vi "My_DHT11_Labview2.vi"() -> ()   [LabVIEW 2024]
uses:
  <vilib>/Instr/_visa.llb/VISA Configure Serial Port (Instr).vi
panel:
  out "Boolean 2":bool
  out "Temperature":dbl(graph)
  out "Humidity":dbl(knob) scale=0.0..10.0
  out "Boolean":bool
  out "%":dbl(slide) scale=0.0..100.0 scale format="%%%d"
  out "Hum":string
  out "C":dbl(slide) scale=0.0..100.0
  in  "?":bool
  out "Temp":string
  in  "VISA Arduino Uno":refnum<visa-resource-name>
  # "Monitoring Temp&Hum"
  # "Eng. Yahia Gaddal\ngaddal18@gmail.com"
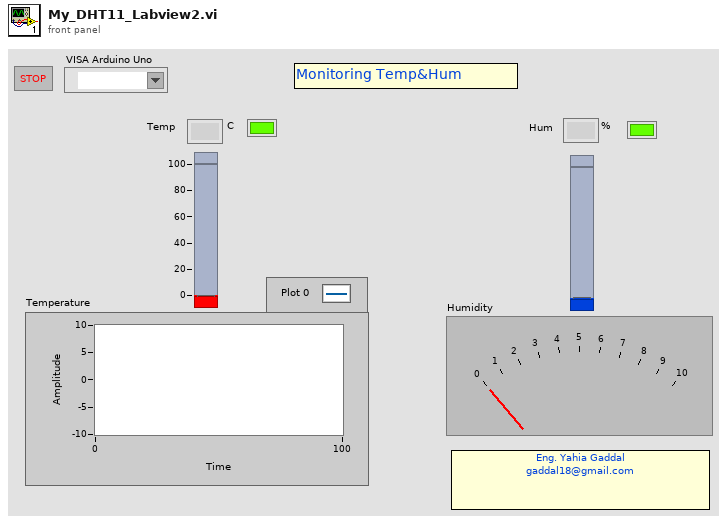
[diagram p1: front panel]
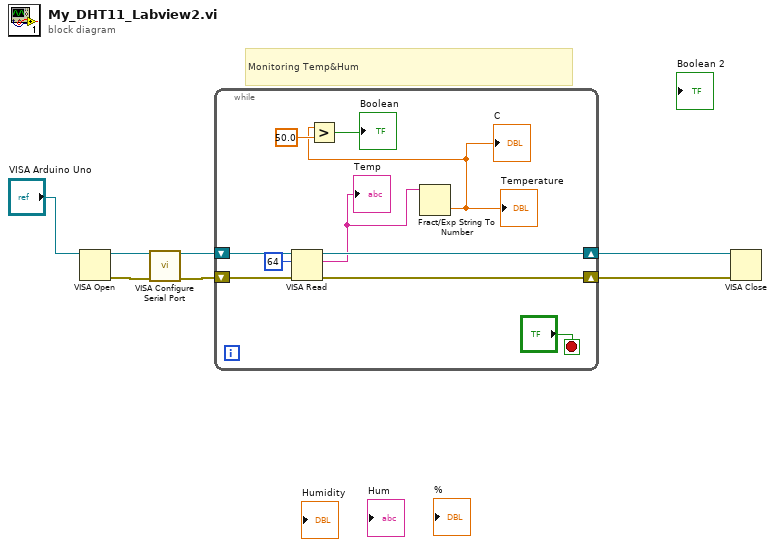
[diagram p0: block diagram]
diagram:
  # "Monitoring Temp&Hum"
  n1 = VISA Open(VISA resource name="VISA Arduino Uno") -> (VISA resource name=w7:refnum<visa-resource-name>, error out=w6:errorcluster)  [unwired: 4 in]
  n2 = call-poly "VISA Configure Serial Port"("VISA resource name"=w7, "error in (no error)"=w6) -> ("VISA resource name out"=w5:refnum<visa-resource-name>, "error out"=w4:errorcluster)  [unwired: 12 in]
  n3 = while {
    shift-right: [w14] -> w3
    shift-left: w5 -> [w17]
    shift-right: [w13] -> w2
    shift-left: w4 -> [w16]
    stop <- "?" stop-if-true
    n4 = VISA Read(VISA resource name=w17, byte count=u32 64, error in (no error)=w16) -> (VISA resource name out=w14:refnum<visa-resource-name>, read buffer=w11:string, error out=w13:errorcluster)  [unwired: 1 out]
    "Temp" <- w11
    n5 = Fract/Exp String To Number(string=w11) -> (number=w8:dbl)  [unwired: 3 in, 1 out]
    "C" <- w8
    "Temperature" <- w8
    n6 = Greater?(x=w8, y=50.0) -> (0:→"Boolean":bool)
  }
  n7 = VISA Close(VISA resource name=w3, error in (no error)=w2) -> ()  [unwired: 1 out]
